vi "Begin.vi"(11 "Image Size":T1=enum."160x120") -> (0 "error out":errorcluster)   [LabVIEW 2015]
doc: "Called before other user functions, this VI is expected to open initial I/O refnums, load in file data, and do all program initialization. Notice that the <B>error out</B> terminal is simply used for data flow. Wiring it to other structures or subVIs ensures that this VI runs first."
uses:
  <vilib>/Rock Robotics/WPI/Camera/WPI_CameraImageSize.ctl
  <vilib>/Rock Robotics/WPI/SafetyOutput/WPI_SafetyOutputConfigMenu.ctl
  <vilib>/Rock Robotics/WPI/DriverStation/WPI_DriverStationRobotMode2.ctl
  <vilib>/Rock Robotics/WPI/Joystick/WPI_JoystickDeviceEnum.ctl
  <vilib>/Rock Robotics/SystemInterfaces/DIO/FPGA_DIOChannel.ctl
  <vilib>/Rock Robotics/SystemInterfaces/DIO/FPGA_DIORelayChannel.ctl
  <vilib>/Rock Robotics/WPI/Solenoid/WPI_SolenoidChannel.ctl
  <vilib>/Rock Robotics/SystemInterfaces/DIO/FPGA_DIOPWMChannel.ctl
  <vilib>/Rock Robotics/SystemInterfaces/Typedef/FPGA_TypedefDigitalModule.ctl
  Robot Global Data.vi
  <vilib>/Rock Robotics/WPI/RobotDrive/WPI_RobotDriveOpen4MotorWithCANJaguar.vi
  <vilib>/Rock Robotics/WPI/Solenoid/WPI_SolenoidOpenDouble.vi
  <vilib>/Rock Robotics/WPI/Compressor/WPI_CompressorGetSetRefNum.vi
  <vilib>/Rock Robotics/WPI/Camera/WPI_CameraWhite Balance Values.ctl
  <vilib>/Rock Robotics/WPI/Camera/WPI_CameraExposure Values.ctl
  <vilib>/Rock Robotics/WPI/Camera/WPI_CameraFrameRate.ctl
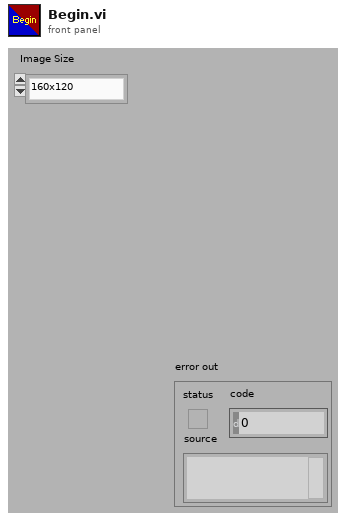
[diagram p1: front panel]
types:
  T1 = typedef "WPI_CameraImageSize.ctl" = enum16{"640x480", "320x240", "160x120"}
  T2 = typedef "FPGA_DIOChannel.ctl" = enum8{"DIO 1", "DIO 2", "DIO 3", "DIO 4", "DIO 5", "DIO 6", "DIO 7", "DIO 8", "DIO 9", "DIO 10", "DIO 11", "DIO 12", "DIO 13", "DIO 14", "Invalid"}
  T3 = typedef "FPGA_TypedefDigitalModule.ctl" = enum16{"Digital Module 1", "Digital Module 2"}
  T4 = typedef "FPGA_DIOPWMChannel.ctl" = enum8{"PWM 1", "PWM 2", "PWM 3", "PWM 4", "PWM 5", "PWM 6", "PWM 7", "PWM 8", "PWM 9", "PWM 10", "Invalid"}
  T5 = typedef "WPI_SolenoidChannel.ctl" = enum8{"Solenoid 1", "Solenoid 2", "Solenoid 3", "Solenoid 4", "Solenoid 5", "Solenoid 6", "Solenoid 7", "Solenoid 8", "Invalid"}
  T6 = typedef "FPGA_DIORelayChannel.ctl" = enum8{"Relay 1", "Relay 2", "Relay 3", "Relay 4", "Relay 5", "Relay 6", "Relay 7", "Relay 8", "Invalid"}
  T7 = typedef "WPI_JoystickDeviceEnum.ctl" = enum16{"USB 0", "USB 1", "USB 2", "USB 3", "USB 4", "USB 5"}
  T8 = typedef "WPI_DriverStationRobotMode2.ctl" = enum16{"Autonomous Disabled", "Autonomous Enabled", "Teleop Disabled", "Teleop Enabled", "Disconnected", "Finish", "Test Disabled", "Test Enabled"}
  T9 = typedef "WPI_SafetyOutputConfigMenu.ctl" = enum16{"Enable", "Disable"}
  T10 = typedef "WPI_CameraFrameRate.ctl" = u32
  T11 = typedef "WPI_CameraExposure Values.ctl" = enum16{"Auto", "Flicker-free 50 Hz", "Flicker-free 60 Hz", "Hold current"}
  T12 = typedef "WPI_CameraWhite Balance Values.ctl" = enum16{"Auto", "Fixed indoor", "Fixed outdoor 1", "Fixed outdoor 2", "Fixed fluorescent 1", "Fixed fluorescent 2", "Hold current"}
  T13 = typedef "WPI_CameraDevRef.ctl" = cluster{"Camera Address":string, "CameraStatus":errorcluster, "Acquire Image Notifier":refnum<notifier>}
  T14 = typedef "WPI_JoystickDevRef.ctl" = cluster{"Device":T7}
  T15 = typedef "WPI_RobotDriveDevRef.ctl" = cluster{"DevStatus":errorcluster, "Motors[]":T16[], "Square Inputs":bool, "Max Output":dbl}
  T16 = typedef "WPI_MotorControlDeviceRef.ctl" = cluster{"DeviceStatus":errorcluster, "Type":enum16{"PWM", "CAN"}, "PWM":cluster{"Digital Module":T3, "PWM Channel":T4, "DeadBand":T17}, "CAN":cluster{"Device Number":u8, "Control Mode":T18, "Semaphore":T19, "Max Vout":dbl}, "Invert":bool, "TransformRef":T20, "InvTransformRef":T20}
  T17 = typedef "WPI_PWMDeadband.ctl" = cluster{"Name":string, "maxPositivePwm":i32, "minPositivePwm":i32, "centerPwm":i32, "maxNegativePwm":i32, "minNegativePwm":i32, "angularRange":u16}
  T18 = typedef "WPI_CANJaguar_ControlMode.ctl" = enum8{"Percent VBus", "Current", "Speed", "Position", "Voltage"}
  T19 = typedef "Semaphore RefNum" = refnum<k1>
  T20 = typedef "WPI_PWMTransform_ConPane.ctl" = refnum<vi>
  T21 = typedef "WPI_RelayDevRef.ctl" = cluster{"DevStatus":errorcluster, "Relay Channel":T6, "Digital Module":T3, "Relay Direction":T22}
  T22 = typedef "WPI_RelayDirection.ctl" = enum16{"Both directions", "Forward only", "Reverse only"}
  T23 = typedef "WPI_SolenoidDevRef.ctl" = cluster{"DevStatus":errorcluster, "Solenoid Module":T24, "Forward Solenoid Channel":T5, "Reverse Solenoid Channel":T5}
  T24 = typedef "FPGA_TypedefSolenoidModule.ctl" = enum16{"Solenoid Module 1", "Solenoid Module 2"}
  T25 = typedef "WPI_DigitalOutputDevRef.ctl" = cluster{"Digital Module":T3, "DIO Channel":T2, "DevStatus":errorcluster}
  T26 = typedef "WPI_DigitalInputDevRef.ctl" = cluster{"DevStatus":errorcluster, "DIO Channel":T2, "Digital Module":T3}
  T27 = typedef "WPI_PWMDeviceRef.ctl" = cluster{"DeviceStatus":errorcluster, "Digital Module":T3, "PWM Channel":T4}
  T28 = typedef "WPI_CompressorDevRef.ctl" = cluster{"DevStatus":errorcluster, "DigitalInputDevRef":T26, "RelayDevRef":T21}
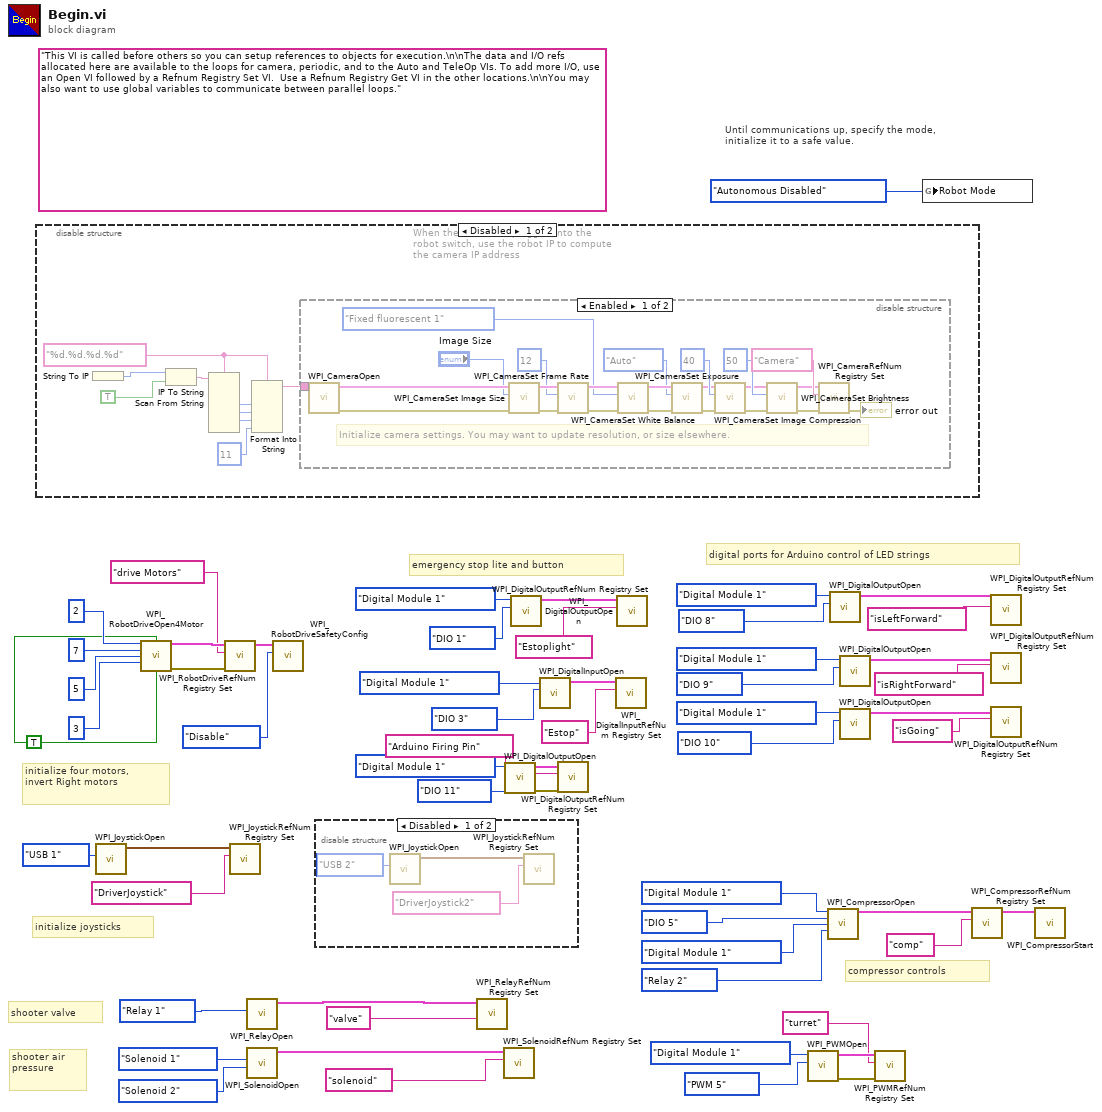
[diagram p0: block diagram]
diagram:
  w45 = TRUE ("Front Right Motor Inverted")
  (unwired) "This VI is called before others so you can setup references to objects for execution.\n\nThe data and I/O refs allocated here are available to the loops for camera, periodic, and to the Auto and TeleOp VIs. To add more I/O, use an Open VI followed by a Refnum Registry Set VI.  Use a Refnum Registry Get VI in the other locations.\n\nYou may also want to use global variables to communicate between parallel loops."
  # "compressor controls"
  # "shooter air\npressure"
  # "shooter valve"
  # "emergency stop lite and button"
  # "digital ports for Arduino control of LED strings"
  # "initialize joysticks"
  # "Until communications up, specify the mode,\ninitialize it to a safe value."
  # "initialize four motors,\ninvert Right motors"
  n1 = disable-structure shown="Disabled" {
    frame Disabled {
      w60 = "%d.%d.%d.%d" ("format string")
      # "When the camera is plugged into the\nrobot switch, use the robot IP to compute\nthe camera IP address"
      n2 = String To IP() -> (0:w67:u32)  [unwired: 1 in]
      n3 = IP To String(1:TRUE ("dot notation? (F)"), 2:w67) -> (0:w65:string)
      n4 = Scan From String(format string=w60, input string=w65) -> (output 1=w64:i32, output 2=w63:i32, output 3=w62:i32)  [unwired: 7 in, 3 out]
      n5 = Format Into String(format string=w60, w64, w63, w62, 11 ("Compression")) -> (resulting string=w59:string)  [unwired: 2 in, 1 out]
      n6 = disable-structure shown="Enabled" {
        disable-tunnel: w59 -> [w69 _]
        frame Enabled {
          # "Initialize camera settings. You may want to update resolution, or size elsewhere."
          n7 = call <vilib>:"WPI_CameraOpen.vi"("Camera Address"=w69) -> ("error out"=w81:errorcluster, "CameraDevRef"=w82:T13)  [unwired: 1 in, 8 out]
          n8 = call <vilib>:"WPI_CameraSet Image Size.vi"("error in (no error)"=w81, "Image Size"="Image Size", "CameraDevRef"=w82) -> ("error out"=w80:errorcluster, "CameraDevRef Out"=w83:T13)  [unwired: 7 out]
          n9 = call <vilib>:"WPI_CameraSet Frame Rate.vi"("error in (no error)"=w80, "Frame Rate (fps)"=T10 12, "CameraDevRef"=w83) -> ("error out"=w79:errorcluster, "CameraDevRef Out"=w85:T13)  [unwired: 7 out]
          n10 = call <vilib>:"WPI_CameraSet White Balance.vi"("error in (no error)"=w79, "White Balance"=WPI_CameraWhite_Balance_Values."Fixed fluorescent 1", "CameraDevRef"=w85) -> ("error out"=w78:errorcluster, "CameraDevRef Out"=w84:T13)  [unwired: 7 out]
          n11 = call <vilib>:"WPI_CameraSet Exposure.vi"("error in (no error)"=w78, "Exposure"=WPI_CameraExposure_Values."Auto", "CameraDevRef"=w84) -> ("error out"=w77:errorcluster, "CameraDevRef Out"=w87:T13)  [unwired: 7 out]
          n12 = call <vilib>:"WPI_CameraSet Image Compression.vi"("error in (no error)"=w77, "Compression"=40, "CameraDevRef"=w87) -> ("error out"=w76:errorcluster, "CameraDevRef Out"=w86:T13)  [unwired: 7 out]
          n13 = call <vilib>:"WPI_CameraSet Brightness.vi"("error in (no error)"=w76, "Brightness"=50, "CameraDevRef"=w86) -> ("error out"=w74:errorcluster, "CameraDevRef Out"=w75:T13)  [unwired: 7 out]
          n14 = call <vilib>:"WPI_CameraRefNum Registry Set.vi"("error in (no error)"=w74, "refnum name"="Camera", "CameraDevRef"=w75) -> ("error out"=→"error out":errorcluster)  [unwired: 8 out]
        }
        frame Disabled {
        }
      }
    }
    frame Enabled {
    }
  }
  n15 = call <vilib>:"WPI_JoystickOpen.vi"("JoystickDevice"=WPI_JoystickDeviceEnum."USB 1") -> ("JoystickDevRef"=w51:T14)  [unwired: 10 in]
  n16 = call-poly <vilib>:"WPI_RobotDriveOpen4Motor.vi"("Rear Left Motor"=u8 2 ("Left Motor"), "Rear Right Motor Inverted"=w45, "Rear Right Motor"=u8 7 ("Right Motor"), "Front Left Motor"=u8 5, "Front Right Motor"=u8 3, "Front Right Motor Inverted"=w45) -> ("RobotDriveDevRef"=w58:T15, "error out"=w56:errorcluster)  [unwired: 8 in]
  n17 = call <vilib>:"WPI_RobotDriveRefNum Registry Set.vi"("error in (no error)"=w56, "refnum name"="drive Motors", "RobotDriveDevRef"=w58) -> ("RobotDriveDevRef"=w55:T15)  [unwired: 8 out]
  n18 = call <vilib>:"WPI_JoystickRefNum Registry Set.vi"("refnum name"="DriverJoystick", "JoystickDevRef"=w51) -> ()  [unwired: 8 in, 2 out]
  n19 = call <vilib>:"WPI_RelayOpen.vi"("Relay Channel"=FPGA_DIORelayChannel."Relay 1") -> ("RelayDevRef"=w18:T21)  [unwired: 9 in, 1 out]
  n20 = call-poly <vilib>:"WPI_SolenoidOpen.vi"("Reverse Solenoid Channel"=WPI_SolenoidChannel."Solenoid 2", "Forward Solenoid Channel"=WPI_SolenoidChannel."Solenoid 1") -> ("SolenoidDevRef"=w19:T23)  [unwired: 8 in, 1 out]
  n21 = call <vilib>:"WPI_RobotDriveSafetyConfig.vi"("mode"=WPI_SafetyOutputConfigMenu."Disable", "RobotDriveDevRef"=w55) -> ()  [unwired: 8 in, 2 out]
  n22 = disable-structure shown="Disabled" {
    frame Disabled {
      n23 = call <vilib>:"WPI_JoystickOpen.vi"("JoystickDevice"=WPI_JoystickDeviceEnum."USB 2") -> ("JoystickDevRef"=w92:T14)  [unwired: 10 in]
      n24 = call <vilib>:"WPI_JoystickRefNum Registry Set.vi"("refnum name"="DriverJoystick2", "JoystickDevRef"=w92) -> ()  [unwired: 8 in, 2 out]
    }
    frame Enabled {
    }
  }
  n25 = call <vilib>:"WPI_RelayRefNum Registry Set.vi"("refnum name"="valve", "RelayDevRef"=w18) -> ()  [unwired: 8 in, 2 out]
  n26 = call <vilib>:"WPI_SolenoidRefNum Registry Set.vi"("refnum name"="solenoid", "SolenoidDevRef"=w19) -> ()  [unwired: 8 in, 2 out]
  n27 = call <vilib>:"WPI_DigitalOutputOpen.vi"("DIO Channel"=FPGA_DIOChannel."DIO 11", "Digital Module (Module 1)"=FPGA_TypedefDigitalModule."Digital Module 1") -> ("error out"=w3:errorcluster, "DigitalOutputDevRef"=w2:T25)  [unwired: 8 in]
  n28 = call <vilib>:"WPI_DigitalOutputOpen.vi"("DIO Channel"=FPGA_DIOChannel."DIO 1", "Digital Module (Module 1)"=FPGA_TypedefDigitalModule."Digital Module 1") -> ("DigitalOutputDevRef"=w33:T25)  [unwired: 8 in, 1 out]
  n29 = call <vilib>:"WPI_DigitalInputOpen.vi"("DIO Channel"=FPGA_DIOChannel."DIO 3", "Digital Module (Module 1)"=FPGA_TypedefDigitalModule."Digital Module 1") -> ("DigitalInputDevRef"=w30:T26)  [unwired: 8 in, 1 out]
  n30 = call <vilib>:"WPI_DigitalOutputRefNum Registry Set.vi"("error in (no error)"=w3, "refnum name"="Arduino Firing Pin", "DigitalOutputDevRef"=w2) -> ()  [unwired: 7 in, 2 out]
  n31 = call <vilib>:"WPI_DigitalInputRefNum Registry Set.vi"("refnum name"="Estop", "DigitalInputDevRef"=w30) -> ()  [unwired: 8 in, 2 out]
  n32 = call <vilib>:"WPI_DigitalOutputRefNum Registry Set.vi"("refnum name"="Estoplight", "DigitalOutputDevRef"=w33) -> ()  [unwired: 8 in, 2 out]
  n33 = call <vilib>:"WPI_PWMOpen.vi"("PWM Channel"=FPGA_DIOPWMChannel."PWM 5", "Digital Module (Module 1)"=FPGA_TypedefDigitalModule."Digital Module 1") -> ("error out"=w14:errorcluster, "PWMDeviceRef"=w15:T27)  [unwired: 8 in]
  n34 = call <vilib>:"WPI_CompressorOpen.vi"("Pressure Switch Digital Module (Module 1)"=FPGA_TypedefDigitalModule."Digital Module 1", "Pressure Switch DIO Channel"=FPGA_DIOChannel."DIO 5", "Relay Digital Module (Module 1)"=FPGA_TypedefDigitalModule."Digital Module 1", "Relay Channel"=FPGA_DIORelayChannel."Relay 2") -> ("CompressorDevRef"=w10:T28)  [unwired: 10 in, 1 out]
  n35 = call <vilib>:"WPI_DigitalOutputOpen.vi"("DIO Channel"=FPGA_DIOChannel."DIO 8", "Digital Module (Module 1)"=FPGA_TypedefDigitalModule."Digital Module 1") -> ("DigitalOutputDevRef"=w37:T25)  [unwired: 8 in, 1 out]
  n36 = call <vilib>:"WPI_DigitalOutputOpen.vi"("DIO Channel"=FPGA_DIOChannel."DIO 9", "Digital Module (Module 1)"=FPGA_TypedefDigitalModule."Digital Module 1") -> ("DigitalOutputDevRef"=w38:T25)  [unwired: 8 in, 1 out]
  n37 = call <vilib>:"WPI_DigitalOutputOpen.vi"("DIO Channel"=FPGA_DIOChannel."DIO 10", "Digital Module (Module 1)"=FPGA_TypedefDigitalModule."Digital Module 1") -> ("DigitalOutputDevRef"=w6:T25)  [unwired: 8 in, 1 out]
  n38 = call <vilib>:"WPI_PWMRefNum Registry Set.vi"("error in (no error)"=w14, "refnum name"="turret", "PWMDeviceRef"=w15) -> ()  [unwired: 7 in, 2 out]
  n39 = global write "Robot Global Data.vi" "Robot Mode"(WPI_DriverStationRobotMode2."Autonomous Disabled" ("Robot Mode")) -> ()
  n40 = call <vilib>:"WPI_CompressorRefNum Registry Set.vi"("refnum name"="comp", "CompressorDevRef"=w10) -> ("CompressorDevRef"=w9:T28)  [unwired: 8 in, 1 out]
  n41 = call <vilib>:"WPI_DigitalOutputRefNum Registry Set.vi"("refnum name"="isLeftForward", "DigitalOutputDevRef"=w37) -> ()  [unwired: 8 in, 2 out]
  n42 = call <vilib>:"WPI_DigitalOutputRefNum Registry Set.vi"("refnum name"="isRightForward", "DigitalOutputDevRef"=w38) -> ()  [unwired: 8 in, 2 out]
  n43 = call <vilib>:"WPI_DigitalOutputRefNum Registry Set.vi"("refnum name"="isGoing", "DigitalOutputDevRef"=w6) -> ()  [unwired: 8 in, 2 out]
  n44 = call <vilib>:"WPI_CompressorStart.vi"("CompressorDevRef"=w9) -> ()  [unwired: 9 in, 2 out]
